vi "Get Inbound Events.vi"(8 "error in (no error)":errorcluster, 11 "Value Editor Base in":refnum<class "Value Editor Base.lvclass">) -> (0 "error out":errorcluster, 2 "Inbound Events":T1, 3 "Value Editor Base out":refnum<class "Value Editor Base.lvclass">)   [LabVIEW 2020, in "Value Editor Base.lvclass"]
uses:
  Value Editor Base.lvclass
  Value Editor Base.lvclass/Value Editor Base.ctl
  Terminal Direction.ctl
  FlexBlocks.lvlib
  Value Mode.ctl
  Special Terminal.ctl
  Type Descriptor.ctl
  Update Type Data.ctl
  Terminal Mode.ctl
  Terminal Mode Data.ctl
  Update Value Data.ctl
  Inbound Events.ctl
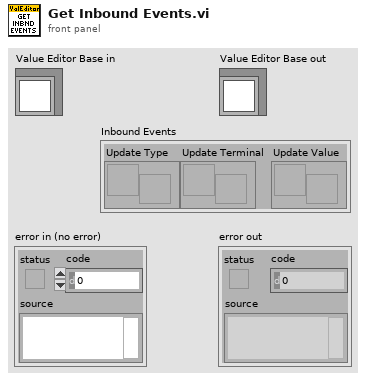
[diagram p1: front panel]
types:
  T1 = typedef "Value Editor Base.lvclass/Inbound Events.ctl" = cluster{"Update Type":refnum<user-event>, "Update Terminal":refnum<user-event>, "Update Value":refnum<user-event>}
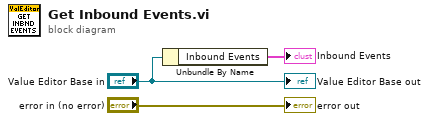
[diagram p0: block diagram]
diagram:
  n1 = Unbundle By Name("Value Editor Base in") -> ("Inbound Events"=→"Inbound Events":T1)
  "error out" <- "error in (no error)"
  "Value Editor Base out" <- "Value Editor Base in"
